vi "USB4704 #0 V1.vi"(6 "Time out":i32, 9 "Samples":i32, 10 "Rate":i32, 11 "start/stop":bool) -> (0 "error out":errorcluster, 3 "data out(DDT)":dynamicdata(waveform))   [LabVIEW 2013]
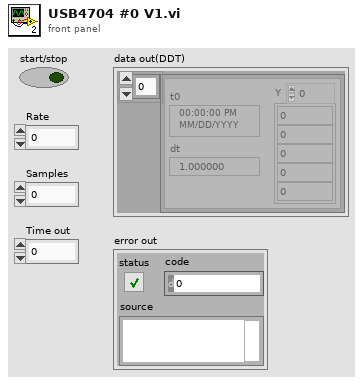
[diagram p1: front panel]
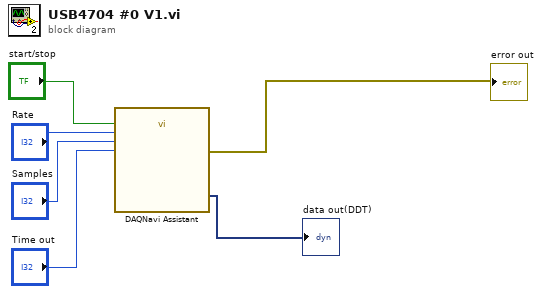
[diagram p0: block diagram]
diagram:
  n1 = call "DAQNavi Assistant"("stop(true)"="start/stop", "conversion rate(Hz)"="Rate", "samples"="Samples", "time out(10s)"="Time out") -> ("error out"=→"error out":errorcluster, "data out(DDT)"=→"data out(DDT)":dynamicdata)  [unwired: 22 in]
